vi "WRITE NEO values.vi"(8 "error in (no error)":errorcluster, 10 "MotorControlDevRef":T1, 11 "RefName":string) -> (0 "error out":errorcluster)   [LabVIEW 2020]
uses:
  <vilib>/Rock Robotics/WPI/MotorControl/WPI_MotorControlDeviceRef.ctl
  <vilib>/Rock Robotics/WPI/MotorControl/WPI_MotorControlType.ctl
  <vilib>/Rock Robotics/SystemInterfaces/DIO/FPGA_DIOPWMChannel.ctl
  <vilib>/Rock Robotics/WPI/PWM/WPI_PWMDeadband.ctl
  <vilib>/Rock Robotics/SystemInterfaces/DIO/FPGA_DIOChannel.ctl
  <vilib>/Rock Robotics/Network Tables/NT Write Boolean.vi
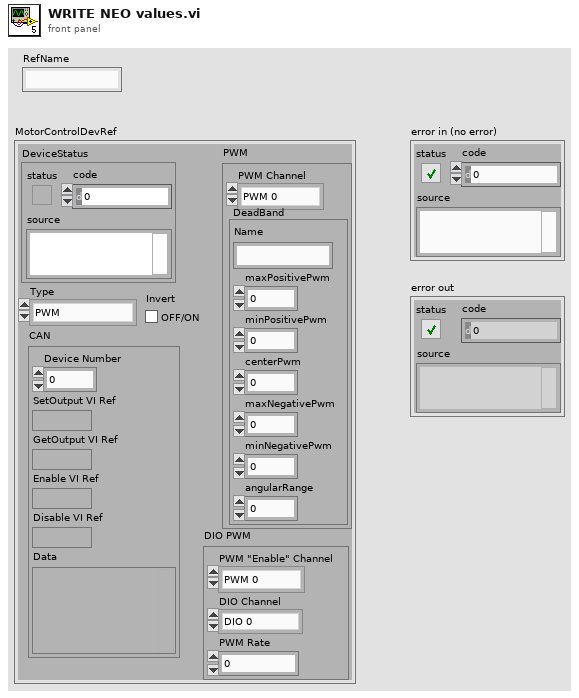
[diagram p1: front panel]
types:
  T1 = typedef "WPI_MotorControlDeviceRef.ctl" = cluster{"DeviceStatus":errorcluster, "Type":T2, "PWM":cluster{"PWM Channel":T3, "DeadBand":T4}, "CAN":cluster{"Device Number":u8, "SetOutput VI Ref":variant, "GetOutput VI Ref":variant, "Enable VI Ref":variant, "Disable VI Ref":variant, "Data":variant}, "Invert":bool, "DIO PWM":cluster{"PWM \"Enable\" Channel":T3, "DIOChannel":T5, "PWM Rate":dbl}}
  T2 = typedef "WPI_MotorControlType.ctl" = enum16{"PWM", "CAN", "DIO PWM"}
  T3 = typedef "FPGA_DIOPWMChannel.ctl" = enum8{"PWM 0", "PWM 1", "PWM 2", "PWM 3", "PWM 4", "PWM 5", "PWM 6", "PWM 7", "PWM 8", "PWM 9", "PWM MXP 0", "PWM MXP 1", "PWM MXP 2", "PWM MXP 3", "PWM MXP 4", "PWM MXP 5", "PWM MXP 6", "PWM MXP 7", "PWM MXP 8", "PWM MXP 9", "Invalid"}
  T4 = typedef "WPI_PWMDeadband.ctl" = cluster{"Name":string, "maxPositivePwm":i32, "minPositivePwm":i32, "centerPwm":i32, "maxNegativePwm":i32, "minNegativePwm":i32, "angularRange":u16}
  T5 = typedef "FPGA_DIOChannel.ctl" = enum8{"DIO 0", "DIO 1", "DIO 2", "DIO 3", "DIO 4", "DIO 5", "DIO 6", "DIO 7", "DIO 8", "DIO 9", "DIO MXP 0", "DIO MXP 1", "DIO MXP 2", "DIO MXP 3", "DIO MXP 4", "DIO MXP 5", "DIO MXP 6", "DIO MXP 7", "DIO MXP 8", "DIO MXP 9", "DIO MXP 10", "DIO MXP 11", "DIO MXP 12", "DIO MXP 13", "DIO MXP 14", "DIO MXP 15", "SPI Port CS1", "SPI Port CS2", "SPI Port CS3", "SPI Port MISO", "SPI Port MOSI", "Invalid"}
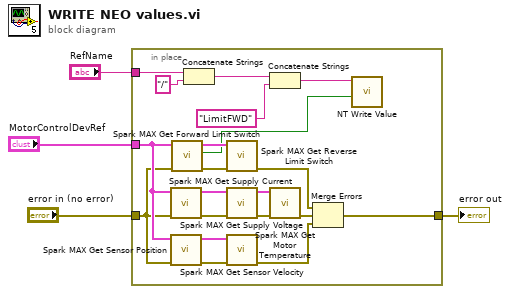
[diagram p0: block diagram]
diagram:
  n1 = in-place {
    in-place-border: "MotorControlDevRef" -> [w16]
    in-place-border: [w14] -> w2
    in-place-border: "error in (no error)" -> [w13]
    in-place-border: "RefName" -> [w10]
    n2 = call <vilib>:"Spark MAX Get Supply Current.vi"("error in (no error)"=w13, "MotorControlDevRef in"=w16) -> ("error out"=w22:errorcluster, "MotorControlDevRef out"=w18:T1)  [unwired: 6 in, 2 out]
    n3 = call <vilib>:"Spark MAX Get Sensor Position.vi"("error in (no error)"=w13, "MotorControlDevRef in"=w16) -> ("error out"=w24:errorcluster, "MotorControlDevRef out"=w19:T1)  [unwired: 6 in, 2 out]
    n4 = call <vilib>:"Spark MAX Get Forward Limit Switch.vi"("error in (no error)"=w13, "MotorControlDevRef in"=w16) -> ("error out"=w23:errorcluster, "Hard Limit Fwd"=w6:bool, "MotorControlDevRef out"=w20:T1)  [unwired: 6 in, 1 out]
    n5 = Concatenate Strings(w10, "/" ("string")) -> (w8:string)
    n6 = call <vilib>:"Spark MAX Get Reverse Limit Switch.vi"("error in (no error)"=w23, "MotorControlDevRef in"=w20) -> ("error out"=w12:errorcluster)  [unwired: 6 in, 3 out]
    n7 = call <vilib>:"Spark MAX Get Supply Voltage.vi"("error in (no error)"=w22, "MotorControlDevRef in"=w18) -> ("error out"=w21:errorcluster, "MotorControlDevRef out"=w17:T1)  [unwired: 6 in, 2 out]
    n8 = call <vilib>:"Spark MAX Get Sensor Velocity.vi"("error in (no error)"=w24, "MotorControlDevRef in"=w19) -> ("error out"=w15:errorcluster)  [unwired: 6 in, 3 out]
    n9 = Concatenate Strings(w8, "LimitFWD" ("string")) -> (w7:string)
    n10 = call <vilib>:"Spark MAX Get Motor Temperature.vi"("error in (no error)"=w21, "MotorControlDevRef in"=w17) -> ("error out"=w11:errorcluster)  [unwired: 6 in, 3 out]
    n11 = Merge Errors(w12, w11, w15) -> (w14:errorcluster)
    n12 = call-poly <vilib>:"NT Write Value.vi"("Boolean"=w6, "Name"=w7) -> ()  [unwired: 9 in, 1 out]
  }
  "error out" <- w2
